vi "writeArrayToFile.vi"(3 "error in (no error)":errorcluster, 4 "output file":path, 5 "array":dbl[][](array[numeric]) format="%_5f") -> (0 "error out":errorcluster)   [LabVIEW 2014, in "Array.lvlib"]
uses:
  Array.lvlib
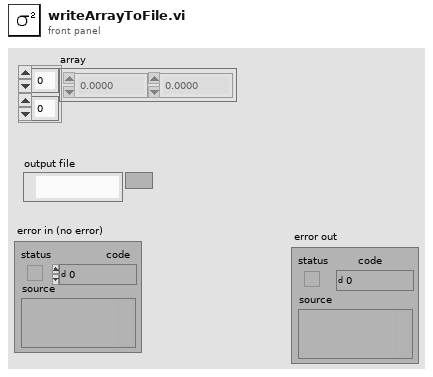
[diagram p1: front panel]
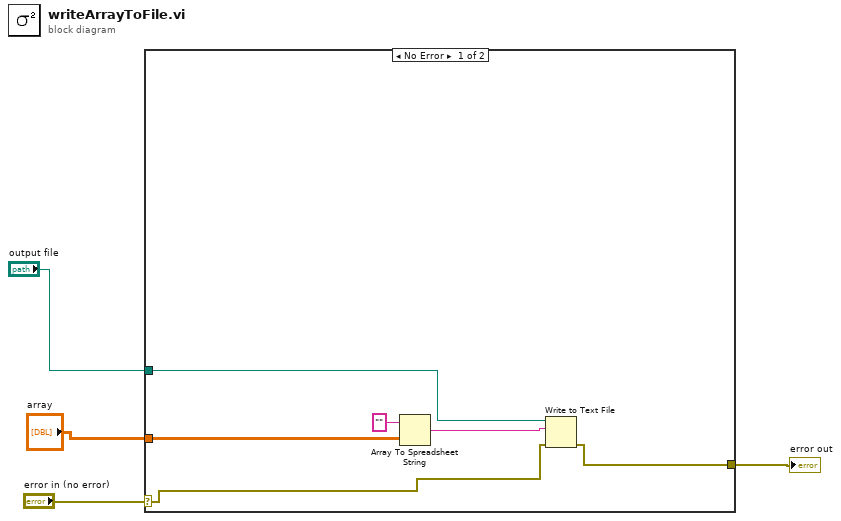
[diagram p0: block diagram]
diagram:
  n1 = case shown="No Error" "error in (no error)" {
    selector: "error in (no error)" -> [w6 w11]
    tunnel: [w7 w11] -> w3
    tunnel: "output file" -> [w8 _]
    tunnel: "array" -> [w5 _]
    frame No Error {
      n2 = Array To Spreadsheet String(array=w5, 3:"" ("format string")) -> (spreadsheet string=w10:string)  [unwired: 1 in]
      n3 = Write to Text File(file (use dialog)=w8, text=w10, error in=w6) -> (error out=w7:errorcluster)  [unwired: 1 in, 2 out]
    }
    frame Error {
    }
  }
  "error out" <- w3
